vi "Msgbox - Status.vi"(8 "Error In":errorcluster) -> (0 "Error Out":errorcluster)   [LabVIEW 2013]
uses:
  Controls/Msgbox Timer Cluster.ctl
  <vilib>/Utility/miscctls.llb/LVPointTypeDef.ctl
panel:
  out "i":i32
  out "Target seconds":i32
  out "Stop":bool
  out "Slide":u8(slide) scale=0.0..100.0
  out "String":string
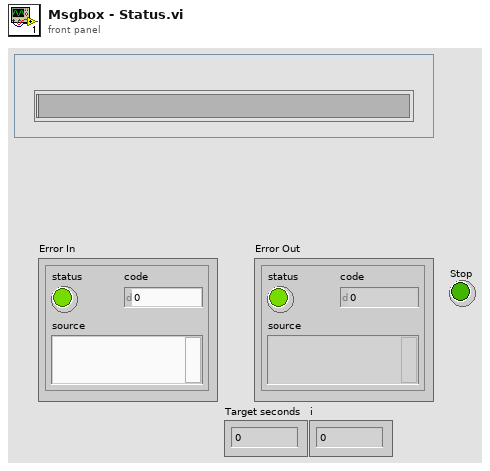
[diagram p1: front panel]
types:
  T1 = typedef "Msgbox Timer Cluster.ctl" = cluster{"Show":bool, "Priority":i32, "Message":string, "seconds":i32}
  T2 = typedef "LVPointTypeDef.ctl" = cluster{"Horizontal":i16, "Vertical":i16}
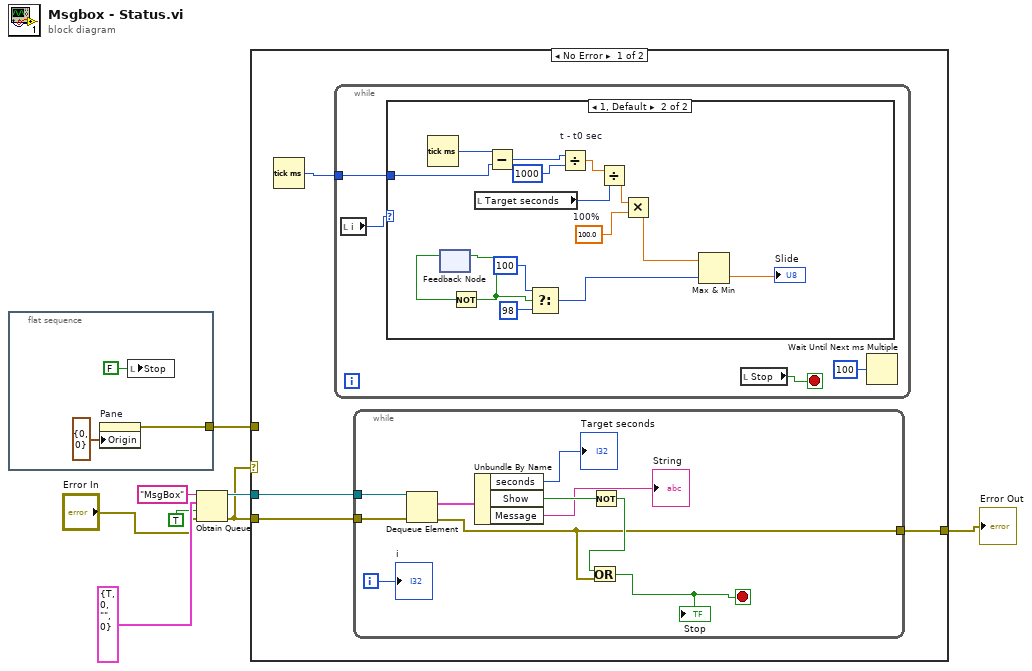
[diagram p0: block diagram]
diagram:
  n1 = flat-sequence {
    tunnel: [w10] -> w1
    frame #0 {
      n2 = property on="Pane" class="Pane"("Origin"=T2 {"Horizontal"=0, "Vertical"=0}) -> (error out=w10:errorcluster)  [unwired: 2 in, 1 out]
      n3 = local write "Stop"(FALSE ("Stop")) -> ()
    }
  }
  n4 = Obtain Queue(name (unnamed)="MsgBox", element data type=T1 {"Show"=TRUE, "Priority"=0, "Message"="", "seconds"=0}, create if not found? (T)=TRUE, error in (no error)="Error In") -> (queue out=w5:refnum<queue>, error out=w4:errorcluster)  [unwired: 1 in, 1 out]
  n5 = case shown="No Error" w4 {
    tunnel: w5 -> [w15 _]
    tunnel: w4 -> [w14 w45]
    tunnel: [w13 w45] -> w2
    tunnel: w1 -> [_ _]
    frame No Error {
      n6 = Tick Count (ms)() -> (millisecond timer value=w12:u32)
      n7 = while {
        tunnel: w12 -> [w18]
        stop <- w19 stop-if-true
        n8 = local read "i"() -> (w16:i32)
        n9 = case shown="1, Default" w16 {
          tunnel: w18 -> [_ w28]
          frame 0 {
            # "Bottom Queue just started"
          }
          frame 1, Default {
            w23 = 100.0  # 100%
            n10 = Tick Count (ms)() -> (millisecond timer value=w29:u32)
            n11 = feedback #1() -> (w34:bool)  [unwired: 1 in]
            n12 = Not(x=w34) -> (.not. x?=w33:bool)
            n13 = feedback-in #1(w33) -> ()
            n14 = local read "Target seconds"() -> (w26:i32)
            n15 = Subtract(x=w29, y=w28) -> (x-y=w22:u32)
            n16 = Select(t=100 ("y"), s=w33, f=98 ("y")) -> (s? t:f=w30:i32)
            n17 = Divide "t - t0 sec"(x=w22, y=u32 1000 ("x")) -> (x/y=w27:dbl)
            n18 = Divide(x=w27, y=w26) -> (x/y=w25:dbl)
            n19 = Multiply(x=w25, y=w23) -> (x*y=w24:dbl)
            n20 = Max & Min(x=w24, y=w30) -> (min(x,y)=→"Slide":dbl)  [unwired: 1 out]
          }
        }
        n21 = local read "Stop"() -> (w19:bool)
        n22 = Wait Until Next ms Multiple(millisecond multiple=u32 100) -> ()  [unwired: 1 out]
      }
      n23 = while {
        tunnel: w15 -> [w44]
        tunnel: w14 -> [w43]
        tunnel: [w38] -> w13
        i -> [w35]
        stop <- w37 stop-if-true
        n24 = Dequeue Element(queue=w44, error in (no error)=w43) -> (element=w42:T1, error out=w38:errorcluster)  [unwired: 1 in, 2 out]
        n25 = Unbundle By Name(w42) -> ("seconds"=→"Target seconds":i32, "Show"=w41:bool, "Message"=→"String":string)
        n26 = Not(x=w41) -> (.not. x?=w39:bool)
        n27 = Or(x=w39, y=w38) -> (x .or. y?=w37:bool)
        "Stop" <- w37
        "i" <- w35
      }
    }
    frame Error {
    }
  }
  "Error Out" <- w2
